vi "Vision_Processing_L_R9.vi"(0 "Current State":T2(ring), 1 "Image Dst":T6=refnum, 2 "Inpute Image":T6=refnum, 3 "Startup Flag":bool, 5 "Current ROI Descriptor":T11={"Global Rectangle"=[0, 0, 320, 220], "Contours"=[{"ID"=enum."External", "Type"=12, "Coordinates"=[0, 0, 320, 220, 0]}]} {"Contours"."Type" items=["No Selection", "Point", "Line", "Rectangle", "Oval", "Polygon", "Freehand Region", "Annulus", "Unused2", "Unused3", "Broken Line", "Freehand Line", "Rotated Rectangle"]}, 6 "Avg Score - Last":dbl=997.186962890625, 7 "error in (no error)":errorcluster, 8 "Current Settings":T9={"Curve Parameters"={"Extraction Mode"=1, "Edge Threshold"=150, "Edge Filter Size"=0, "Min Length"=15, "Row Search Step Size"=10, "Col Search Step Size"=10, "Max Endpoint Gap"=2, "Closed"=TRUE, "Subpixel"=TRUE}, "Match Mode"={"Rotation"=TRUE, "Scale"=TRUE, "Occlusion"=TRUE, "Reserved"=FALSE, "Reserved"=FALSE, "Reserved"=FALSE}, "Range Settings"=[{"Match Constraints"=0, "Min"=-5.0, "Max"=5.0}, {"Match Constraints"=1, "Min"=149.98635845184327, "Max"=172.71047382354737}, {"Match Constraints"=2, "Min"=0.0, "Max"=20.0}], "Number of Matches"=1, "Minimum Match Score"=900.0, "SubPixel Accuracy"=TRUE, "Adv. Geometric Match Options 2"=[{"Setup Data Item"=20, "Item Value"=0.0}, {"Setup Data Item"=22, "Item Value"=1.0}]} {"Curve Parameters"."Extraction Mode" items=["Normal", "Uniform Regions"]; "Curve Parameters"."Edge Filter Size" items=["Fine", "Normal", "Contour Tracing"]; "Curve Parameters"."Max Endpoint Gap" min=0; "Curve Parameters"."Col Search Step Size" min=1 max=255 step=1; "Curve Parameters"."Row Search Step Size" min=1 max=255 step=1; "Curve Parameters"."Min Length" min=0; "Curve Parameters"."Edge Threshold" min=1 max=350 step=1; "Range Settings"."Max" format="%.2f"; "Range Settings"."Min" format="%.2f"; "Range Settings"."Match Constraints" items=["Rotation Angle (degrees)", "Scale Factor (%)", "Occlusion (%)"]; "Adv. Geometric Match Options 2"."Setup Data Item" items=["Curve Extraction Mode", "Curve Edge Threshold", "Curve Edge Filter Size", "Min Curve Length", "Curve Row Search Step Size", "Curve Col Search Step Size", "Curve Max Endpoint Gap", "Extract Closed Curves", "Enable Subpixel Curve Extraction", "Enable Correlation Score", "Enable Subpixel Accuracy", "Subpixel Iterations", "Subpixel Tolerance", "Initial Match List Length", "Enable Target Template Curve Score", "Min Match Separation Distance", "Min Match Separation Angle", "Min Match Separation Scale", "Max Match Overlap", "Enable Coarse Result", "Enable Calibration Support", "Enable Contrast Reversal", "Search Strategy", "Refinement Match Factor", "Subpixel Match Factor"]}, 9 "Sub Beacon Search Enable":bool[](array[boolean])=[FALSE, FALSE, FALSE, FALSE, FALSE], 10 "History Data - IN":T5={"Valid Beacon History - in"=[TRUE, TRUE, TRUE, TRUE, TRUE, TRUE, TRUE, TRUE, TRUE, TRUE, TRUE, TRUE, TRUE, TRUE, TRUE, TRUE, TRUE, TRUE, TRUE, TRUE], "Valid Score History"=[996.9906616210938, 997.97216796875, 996.9906616210938, 996.9906616210938, 996.9906616210938, 996.9906616210938, 996.9906616210938, 996.9906616210938, 997.97216796875, 996.9906616210938, 996.9906616210938, 999.7824096679688, 999.7824096679688, 997.97216796875, 999.7824096679688, 999.7824096679688, 999.7824096679688, 999.7824096679688, 999.7824096679688, 999.7824096679688], "Valid Scale History"=[161.25363159179688, 161.6636962890625, 161.2349395751953, 161.27423095703125, 161.31558227539062, 160.97698974609375, 161.38648986816406, 161.37643432617188, 161.23867797851562, 161.21334838867188, 161.1531524658203, 161.44549560546875, 161.62496948242188, 161.1356201171875, 161.96054077148438, 161.54180908203125, 161.68902587890625, 161.53578186035156, 161.7397918701172, 161.8538360595703]} {"Valid Scale History" format="%#_13g"; "Valid Score History" format="%#_13g"}, 13 "Avg Scale - Last":dbl=161.34841613769532, 16 "History Size":i32=20) -> (11 "Avg Scale":dbl=161.34841613769532, 12 "Avg Score":dbl=997.186962890625, 14 "Tracking Info 1":T1={"Tracking Coordinates"={"X"=158.71055603027344, "Y"=95.56468963623047}, "Current Valid"=TRUE, "Current State - Out"=enum."Sub - 2", "Setting Values"={"Min Scale"=149.93676738739015, "Max Scale"=172.64940814971925, "Min Score"=900.0}}, 15 "Next Main ROI Descriptor":T3={"Global Rectangle"=[0, 0, 320, 220], "Contours"=[{"ID"=enum."External", "Type"=12, "Coordinates"=[0, 0, 320, 220, 0]}]} {"Contours"."Type" items=["No Selection", "Point", "Line", "Rectangle", "Oval", "Polygon", "Freehand Region", "Annulus", "Unused2", "Unused3", "Broken Line", "Freehand Line", "Rotated Rectangle"]}, 17 "Beacon - Scales":sgl[](array[numeric])=[163.2041, 163.79373, 0.0, 0.0, 0.0], 18 "History Data - Out":T4={"Valid Beacon History\nOut"=[TRUE, TRUE, TRUE, TRUE, TRUE, TRUE, TRUE, TRUE, TRUE, TRUE, TRUE, TRUE, TRUE, TRUE, TRUE, TRUE, TRUE, TRUE, TRUE, TRUE], "Valid Score History\nOut"=[996.9906616210938, 997.97216796875, 996.9906616210938, 996.9906616210938, 996.9906616210938, 996.9906616210938, 996.9906616210938, 996.9906616210938, 997.97216796875, 996.9906616210938, 996.9906616210938, 999.7824096679688, 999.7824096679688, 997.97216796875, 999.7824096679688, 999.7824096679688, 999.7824096679688, 999.7824096679688, 999.7824096679688, 999.7824096679688], "Valid Scale History\nOut"=[161.25363159179688, 161.6636962890625, 161.2349395751953, 161.27423095703125, 161.31558227539062, 160.97698974609375, 161.38648986816406, 161.37643432617188, 161.23867797851562, 161.21334838867188, 161.1531524658203, 161.44549560546875, 161.62496948242188, 161.1356201171875, 161.96054077148438, 161.54180908203125, 161.68902587890625, 161.53578186035156, 161.7397918701172, 161.8538360595703]} {"Valid Scale History\nOut" format="%#_13g"; "Valid Score History\nOut" format="%#_13g"}, 19 "Y Coordinates":sgl[](array[numeric])=[108.99595, 93.22681, 0.0, 0.0, 0.0], 20 "Beacons Found":bool[](array[boolean])=[TRUE, TRUE, FALSE, FALSE, FALSE], 21 "X Coordinates":sgl[](array[numeric])=[109.63992, 213.33662, 0.0, 0.0, 0.0], 22 "Next State":T2(ring), 23 "Lock Status":bool=TRUE, 24 "Startup Flag - out":bool, 25 "New Settings":T9={"Curve Parameters"={"Extraction Mode"=1, "Edge Threshold"=150, "Edge Filter Size"=0, "Min Length"=15, "Row Search Step Size"=10, "Col Search Step Size"=10, "Max Endpoint Gap"=2, "Closed"=TRUE, "Subpixel"=TRUE}, "Match Mode"={"Rotation"=TRUE, "Scale"=TRUE, "Occlusion"=TRUE, "Reserved"=FALSE, "Reserved"=FALSE, "Reserved"=FALSE}, "Range Settings"=[{"Match Constraints"=0, "Min"=-5.0, "Max"=5.0}, {"Match Constraints"=1, "Min"=149.98635845184327, "Max"=172.71047382354737}, {"Match Constraints"=2, "Min"=0.0, "Max"=20.0}], "Number of Matches"=1, "Minimum Match Score"=900.0, "SubPixel Accuracy"=TRUE, "Adv. Geometric Match Options 2"=[{"Setup Data Item"=20, "Item Value"=0.0}, {"Setup Data Item"=22, "Item Value"=1.0}]} {"Curve Parameters"."Extraction Mode" items=["Normal", "Uniform Regions"]; "Curve Parameters"."Edge Filter Size" items=["Fine", "Normal", "Contour Tracing"]; "Curve Parameters"."Max Endpoint Gap" min=0; "Curve Parameters"."Col Search Step Size" min=1 max=255 step=1; "Curve Parameters"."Row Search Step Size" min=1 max=255 step=1; "Curve Parameters"."Min Length" min=0; "Curve Parameters"."Edge Threshold" min=1 max=350 step=1; "Range Settings"."Max" format="%.2f"; "Range Settings"."Min" format="%.2f"; "Range Settings"."Match Constraints" items=["Rotation Angle (degrees)", "Scale Factor (%)", "Occlusion (%)"]}, 27 "Right Image 2":T6(plugin-control))   [LabVIEW 2015]
uses:
  <vilib>/vision/Image Controls.llb/IMAQ Image.ctl
  <vilib>/vision/Pattern Matching.llb/IMAQ Curve Parameters.ctl
  <vilib>/vision/Pattern Matching.llb/IMAQ Match Range Setting.ctl
panel:
  in  "ROBOT STATE(fwd, bwd, neither)":i32
  out "beacon - Scores":sgl[](array[numeric])=[998.9578, 999.6264, 0.0, 0.0, 0.0]
  in  "Minimum Score\nNormal 5":dbl=850.0
  in  "Minimum Score\nSub 4":dbl=850.0
  in  "Minimum Score\nSub 3":dbl=900.0
  in  "Minimum Score\nSub 2":dbl=900.0
  in  "Sub - 4 - FIle Path":path=path "/home/lvuser/natinst/bin/BeaconTemplates/4_beacons_left.png"
  in  "3 / 2\nTransition Scale":sgl=100.0
  in  "Score\nCushion- tight":dbl=75.0
  in  "Main ROI Decay\nper Fail (Vertical)":i32=5
  in  "ROI_factor(Horiztonal) (2 b)":sgl=2.0
  in  "ROI_factor(vertical) (2 b)":sgl=1.1
  in  "Sub - 2 File Path":path=path "/home/lvuser/natinst/bin/BeaconTemplates/2_beacons_left.png"
  out "Scale Decay \nFactor":dbl=11.36205768585205
  in  "Scale Decay \nFactor":dbl=5.0
  in  "Valid Treshold\nfor Lock":i16=3
  in  "Horiztonall Beacon \nCushion (pixels)":sgl=20.0
  out "New Min Score":dbl=900.0
  out "New Low Scale":dbl=149.98635845184327
  out "New high Scale":dbl=172.71047382354737
  in  "Absolute\nMinimum Score":dbl=800.0
  in  "Absolute\nMaximum Scale":dbl=300.0
  in  "Absolute\nMinimum Scale":dbl=10.0
  in  "Default No Lock\nSetting Values":T10={"Min Scale"=20.0, "Max Scale"=170.0, "Min Score"=800.0}
  in  "Score\nCushion":dbl=75.0
  out "Scale \nCushion":dbl=11.36205768585205
  in  "5 / 4\nTransition Scale":sgl=70.0
  in  "4 / 3\nTransition Scale":sgl=85.0
  in  "Timeout \nThrehsold":i32=1000
  in  "Main ROI Decay\nper Fail (Horiztonal)":i32=25
  in  "ROI_factor(Horiztonal) (4 & 5 b)":sgl=5.0
  in  "ROI_factor(vertical) (4 & 5 b)":sgl=1.5
  in  "ROI_factor(vertical) (3 b)":sgl=2.7
  in  "ROI_factor(Horiztonal) (3 b)":sgl=2.5
  out "Current  Score":sgl=996.99066
  out "Current  Scale":sgl=161.25363
  in  "Fail Count - In":i32
  in  "Sub Beacon Template File Path - ARRAY":path[](array[path])=[path "/home/lvuser/natinst/bin/BeaconTemplates/Sub1.png", path "/home/lvuser/natinst/bin/BeaconTemplates/Sub2.png", path "/home/lvuser/natinst/bin/BeaconTemplates/Sub3.png", path "/home/lvuser/natinst/bin/BeaconTemplates/Sub4.png", path "/home/lvuser/natinst/bin/BeaconTemplates/Sub5.png"]
  in  "Sub - 3 - FIle Path":path=path "/home/lvuser/natinst/bin/BeaconTemplates/3_beacons_left.png"
  in  "Normal - 5 - File Path":path=path "/home/lvuser/natinst/bin/BeaconTemplates/5_beacons.png"
  # "INPUTS"
  # "FILE PATHS"
  # "CONFIG"
  # "OUTPUTS"
  # "************"
  # "Range"
  # "Range"
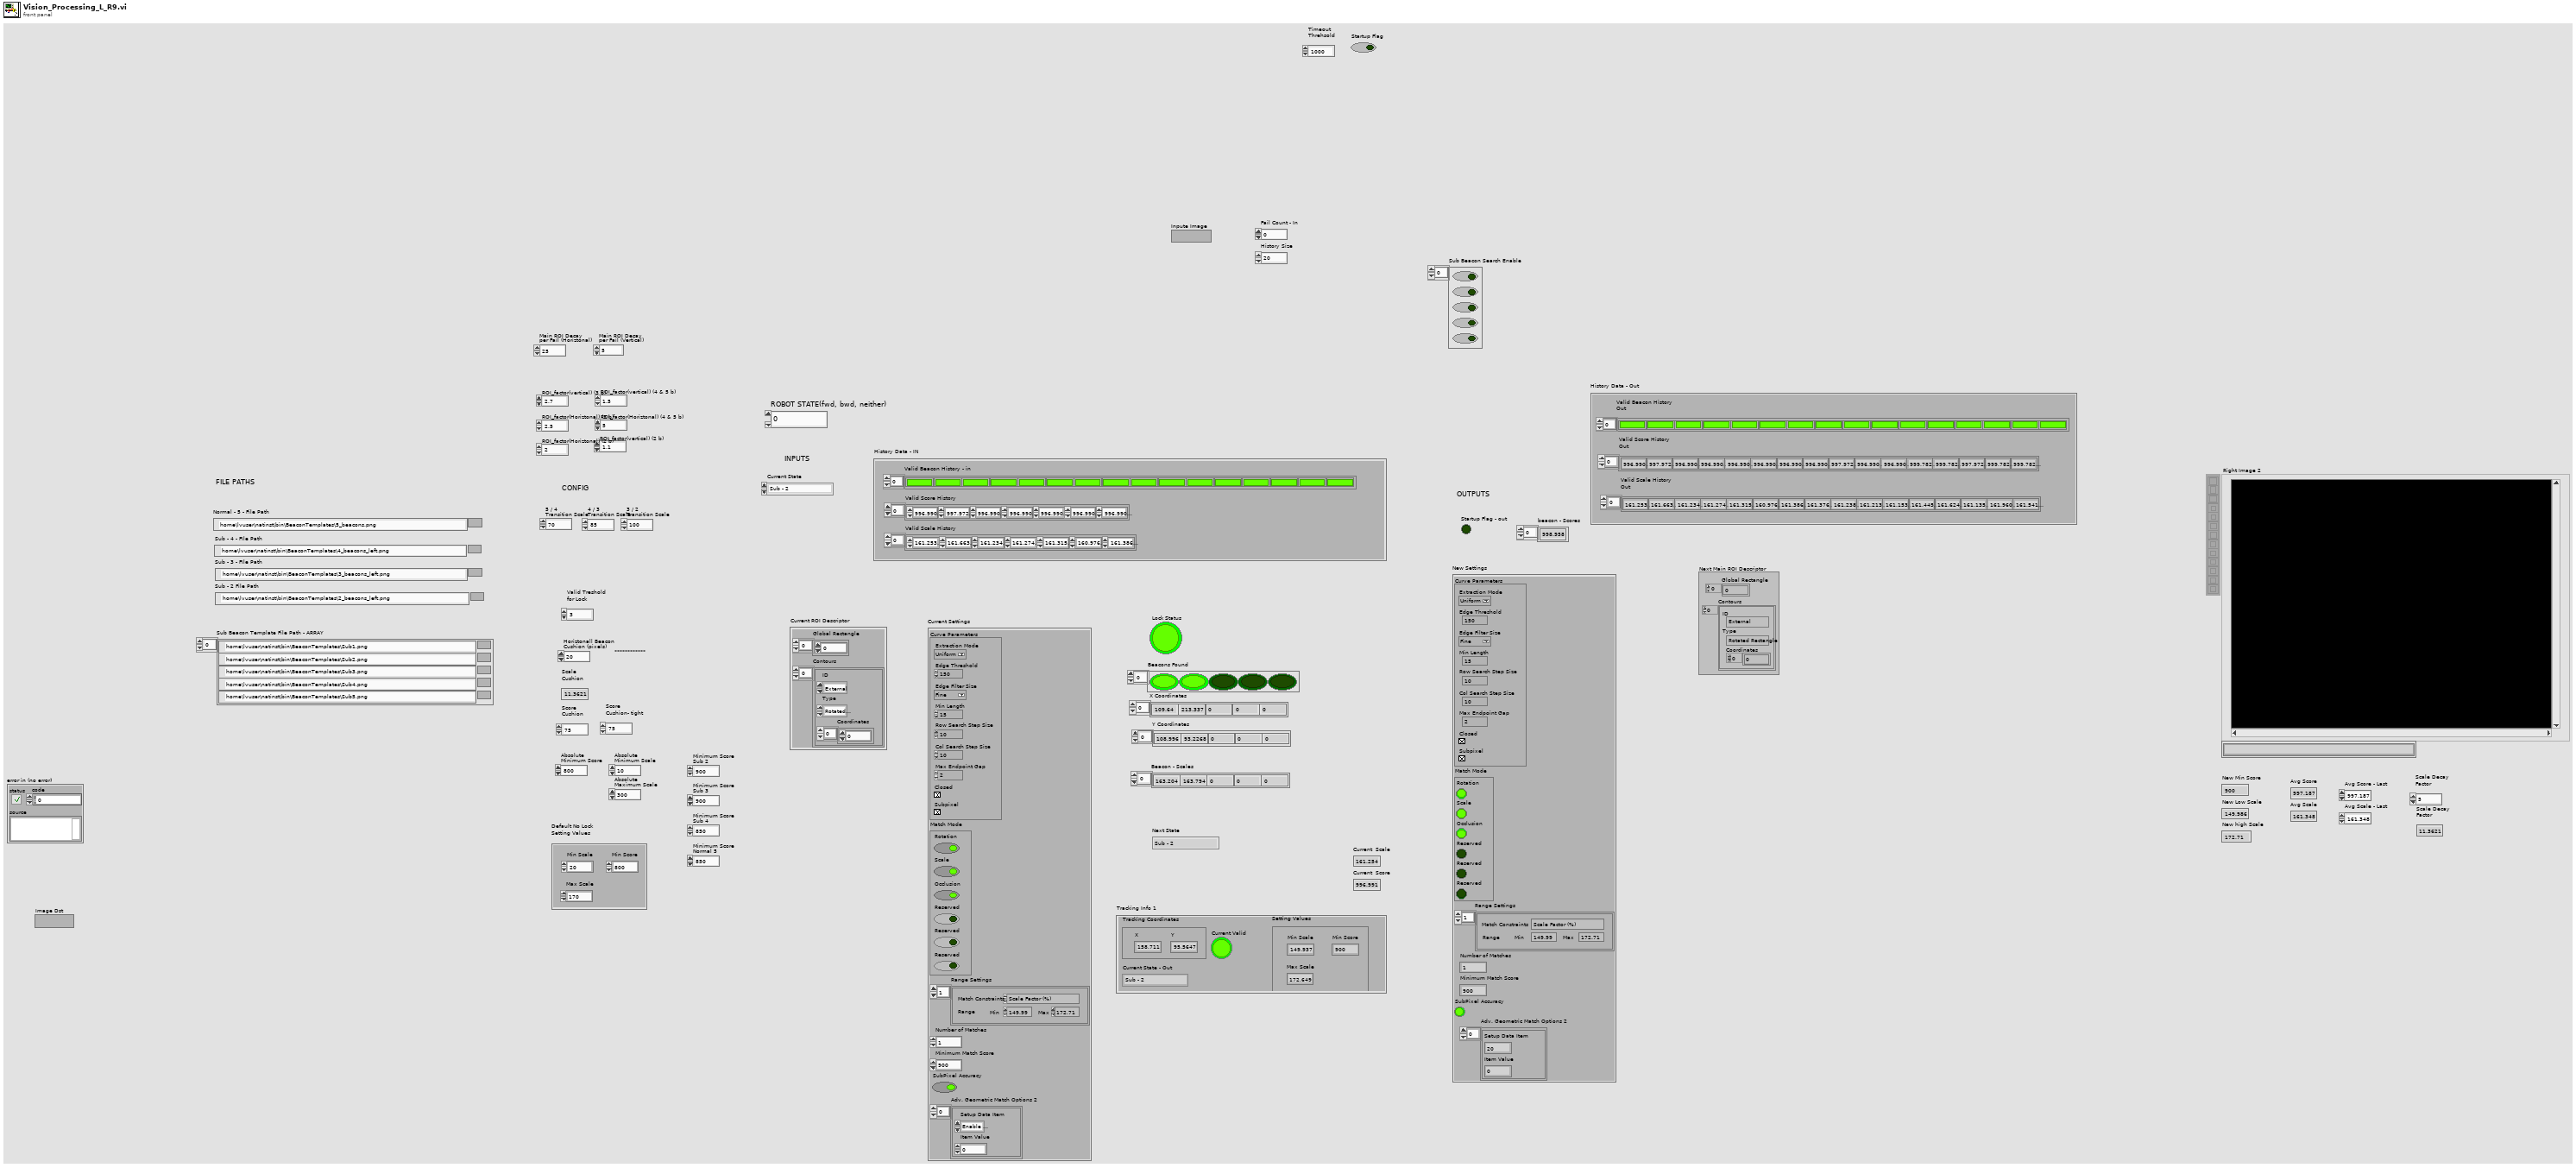
[diagram p1: front panel]
types:
  T1 = cluster{"Tracking Coordinates":cluster{"X":dbl, "Y":dbl}, "Current Valid":bool, "Current State - Out":enum16{"Sub - 2", "Sub - 3", "Sub - 4", "Normal - 5"}, "Setting Values":cluster{"Min Scale":dbl, "Max Scale":dbl, "Min Score":dbl}}
  T2 = enum16{"Sub - 2", "Sub - 3", "Sub - 4", "Normal - 5"}
  T3 = typedef "ROI Descriptor" = cluster{"Global Rectangle":i32[], "Contours":cluster{"ID":enum32{"External", "Internal"}, "Type":u32, "Coordinates":i32[]}[]}
  T4 = cluster{"Valid Beacon History\nOut":bool[], "Valid Score History\nOut":dbl[], "Valid Scale History\nOut":dbl[]}
  T5 = cluster{"Valid Beacon History - in":bool[], "Valid Score History":dbl[], "Valid Scale History":dbl[]}
  T6 = typedef "IMAQ Image.ctl" = refnum<image>
  T7 = typedef "IMAQ Curve Parameters.ctl" = cluster{"Extraction Mode":u32, "Edge Threshold":i32, "Edge Filter Size":u32, "Min Length":i32, "Row Search Step Size":i32, "Col Search Step Size":i32, "Max Endpoint Gap":i32, "Closed":bool, "Subpixel":bool}
  T8 = typedef "IMAQ Match Range Setting.ctl" = cluster{"Match Constraints":u32, "Min":dbl, "Max":dbl}
  T9 = cluster{"Curve Parameters":T7, "Match Mode":cluster{"Rotation":bool, "Scale":bool, "Occlusion":bool, "Reserved":bool, "Reserved":bool, "Reserved":bool}, "Range Settings":T8[], "Number of Matches":i32, "Minimum Match Score":sgl, "SubPixel Accuracy":bool, "Adv. Geometric Match Options 2":cluster{"Setup Data Item":u16, "Item Value":dbl}[]}
  T10 = cluster{"Min Scale":dbl, "Max Scale":dbl, "Min Score":dbl}
  T11 = cluster{"Global Rectangle":i32[], "Contours":cluster{"ID":enum32{"External", "Internal"}, "Type":u32, "Coordinates":i32[]}[]}
  T12 = typedef "IMAQ GM Match Report.ctl" = cluster{"Position":cluster{"x":sgl, "y":sgl}, "Angle":sgl, "Scale":sgl, "Score":sgl, "Bounding Box":cluster{"x":sgl, "y":sgl}[], "Contrast Reversed":bool, "Occlusion %":sgl, "Template Target Curve Score":sgl, "Target Template Curve Score":sgl, "Correlation Score":sgl}
  T13 = cluster{"Matches (Geometric Matching 1)[0]":T12, "Matches (Geometric Matching 1)[1]":T12, "Matches (Geometric Matching 1)[2]":T12, "Matches (Geometric Matching 1)[3]":T12, "Matches (Geometric Matching 1)[4]":T12, "Matches (Geometric Matching 1)[5]":T12, "Matches (Geometric Matching 1)[6]":T12, "Matches (Geometric Matching 1)[7]":T12, "Matches (Geometric Matching 1)[8]":T12}
  T14 = cluster{"Bounding Box[0]":cluster{"x":sgl, "y":sgl}, "Bounding Box[1]":cluster{"x":sgl, "y":sgl}, "Bounding Box[2]":cluster{"x":sgl, "y":sgl}, "Bounding Box[3]":cluster{"x":sgl, "y":sgl}, "Bounding Box[4]":cluster{"x":sgl, "y":sgl}, "Bounding Box[5]":cluster{"x":sgl, "y":sgl}, "Bounding Box[6]":cluster{"x":sgl, "y":sgl}, "Bounding Box[7]":cluster{"x":sgl, "y":sgl}, "Bounding Box[8]":cluster{"x":sgl, "y":sgl}}
  T15 = cluster{"index":u32, "Absolute\nMinimum Scale":dbl, "Absolute\nMaximum Scale":dbl}
  T16 = cluster{"New Low Scale":dbl, "New high Scale":dbl, "New Min Score":dbl}
  T17 = cluster{"Position":cluster{"x":sgl, "y":sgl}, bool, "Current State - Out":enum16{"Sub - 2", "Sub - 3", "Sub - 4", "Normal - 5"}, cluster{"New Low Scale":dbl, "New high Scale":dbl, "New Min Score":dbl}}
  T18 = cluster{"Position":cluster{"x":sgl, "y":sgl}, bool, "Current State":enum16{"Sub - 2", "Sub - 3", "Sub - 4", "Normal - 5"}, cluster{"New Low Scale":dbl, "New high Scale":dbl, "New Min Score":dbl}}
  T19 = typedef "IMAQ Rectangle" = cluster{"Left":i32, "Top":i32, "Right":i32, "Bottom":i32, "Rotation":dbl}
  T20 = cluster{"index":u32, "Min Scale":dbl, "Max Scale":dbl}
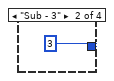
[diagram p3: hidden frame]
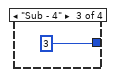
[diagram p4: hidden frame]
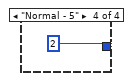
[diagram p5: hidden frame]
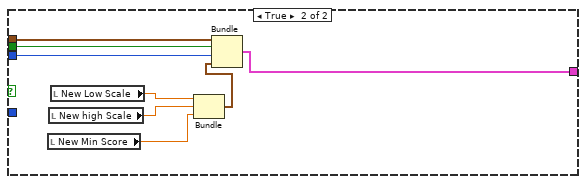
[diagram p6: hidden frame]
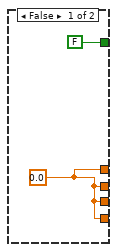
[diagram p7: hidden frame]
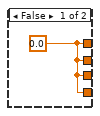
[diagram p8: hidden frame]
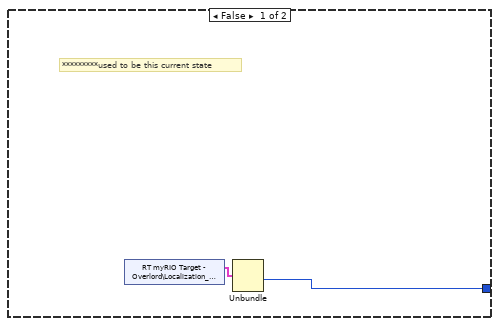
[diagram p12: hidden frame]
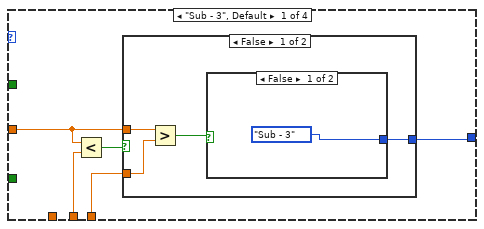
[diagram p13: hidden frame]
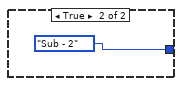
[diagram p14: hidden frame]
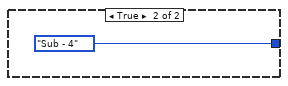
[diagram p15: hidden frame]
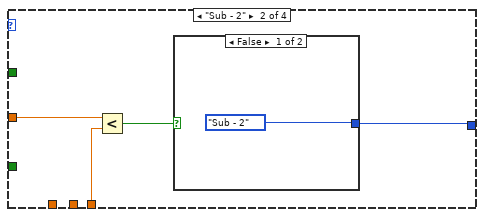
[diagram p16: hidden frame]
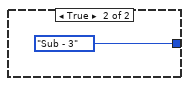
[diagram p17: hidden frame]
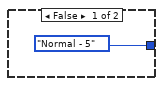
[diagram p18: hidden frame]
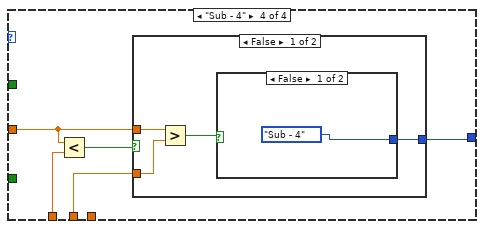
[diagram p19: hidden frame]
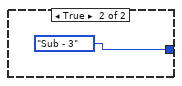
[diagram p20: hidden frame]
diagram:
  (unwired) enum16{"Short Range", "Long Range"}."Short Range"
  # "Next Settings"
  n1 = flat-sequence {
    tunnel: [w8] -> w3
    tunnel: [w7] -> w2
    tunnel: ["Image Dst"] -> w1
    tunnel: w3 -> [w157]
    tunnel: w2 -> [w155]
    tunnel: w1 -> [w156]
    frame #0 {
      # "APPLY FILTERING"
      n2 = call "Camera - Filtering"("Image In"="Inpute Image", "Image Dst"="Image Dst", "error in"="error in (no error)") -> ("Image Out"=w8:T6, "error out"=w7:errorcluster)  [unwired: 23 in]
    }
    frame #1 {
      w38 = u32 1 ("index")
      w119 = u32 1 ("index")
      w140 = u8 5
      # "*************************************************************************************************"
      # "Current Scale"
      # "Lower Scale"
      # "Upper Scale"
      # "Scale"
      # "Start up Template"
      # "Image Lock"
      # "Update Tracking Coordinates"
      # "CURRENT VALID"
      # "*************"
      # "Beacon - Y"
      # "Beacon - X"
      # "Beacons Found"
      # "Build ROI for Individual Beacons Based on Main Bounding Box"
      # "Starting X Lower Bound"
      # "Length of\nIndividual Beacon ROI"
      # "Length of Bounding Box"
      # "Choose ROI Factor based on Next State"
      # "Current Match"
      # "Current ROI"
      # "Image Lock"
      # "Force SR on Startup"
      # "Valid History"
      # "Draw ROI and stuff on outputi mage"
      # "Pull Down Startup IF Already True and Lock\nOtherwise don't update"
      # "Next Settings"
      # "Apply Limits to Settings"
      # "Scale"
      # "Min Score"
      # "Lower Scale"
      # "Upper Scale"
      # "Current Settings"
      # "Current Min\n& Max Scale"
      # "Current Valid"
      # "Update Search Settings"
      # "Update Template State"
      # "Calculate Average Scale/Score"
      # "max avg"
      # "Min Required to use avarage"
      # "Valid  Ccount\n(up to 3)"
      # "****# of previous in history that must be true\nin order for position to be considered \"locked\""
      # "Update Shift Arrays"
      # "# of Beacons Found to be valid"
      # "# of beacons"
      # "Matches"
      # "image out"
      n3 = Select(t=T2."Sub - 2", s="Startup Flag", f="Current State") -> (s? t:f=w47:T2)
      n4 = case shown="\"Sub - 4\"" w47 {
        tunnel: w157 -> [w537 w569 w600 w635]
        tunnel: w156 -> [w536 w568 w599 w634]
        tunnel: "Current ROI Descriptor" -> [w535 w567 w597 w633]
        tunnel: "Current Settings" -> [w534 w566 w596 w632]
        tunnel: [w530 w562 w593 w628] -> w83
        tunnel: [w529 w561 w594 w627] -> w103
        tunnel: [w527 w559 w595 w625] -> w148
        tunnel: w155 -> [_ _ w598 w624]
        tunnel: "Sub Beacon Search Enable" -> [w528 w560 w601 w623]
        tunnel: [sgl 3.0 ("y") sgl 2.0 ("y") 4.0 sgl 5.0 ("y")] -> w153
        tunnel: [w525 w557 w591 w621] -> w152
        tunnel: [2 2 3 4] -> w149
        frame "Sub - 3" {
          n5 = call "Short Range 2"("Image In"=w537, "Image Dst"=w536, "ROI Descriptor (Geometric Matching 1)"=w535, "Settings (Geometric Matching 1)"=w534, "Template File Path (Geometric Matching 1)"="Sub - 3 - FIle Path") -> ("Image Out"=w529:T6, "Matches (Geometric Matching 1)"=w530:T12[], "Number of Matches (Geometric Matching 1)"=w531:i32, "error out"=w525:errorcluster)  [unwired: 19 in]
          n6 = Equal?(x=w531, y=1) -> (x = y?=w532:bool)
          n7 = case shown="True" w532 {
            tunnel: w528 -> [w545 w548]
            tunnel: [w538 w549] -> w527
            frame False {
              w539 = FALSE
              # "F"
              # "No Main Found,\nDon't Search any Subs"
              n8 = Replace Array Subset(array=w545, new element #1=w539, index #1=0 ("y"), new element #2=w539, index #2=1 ("y"), new element #3=w539, index #3=2 ("y"), new element #4=w539, index #4=3 ("y"), new element #5=w539, index #5=4 ("y")) -> (w538:bool[])
            }
            frame True {
              w547 = TRUE
              w546 = FALSE
              n9 = Replace Array Subset(array=w548, new element #1=w547, index #1=0 ("y"), new element #2=w547, index #2=1 ("y"), new element #3=w547, index #3=2 ("y"), new element #4=w546, index #4=3 ("y"), new element #5=w546, index #5=4 ("y")) -> (w549:bool[])
            }
          }
        }
        frame "Sub - 2" {
          n10 = call "Short Range"("Image In"=w569, "Image Dst"=w568, "ROI Descriptor (Geometric Matching 1)"=w567, "Settings (Geometric Matching 1)"=w566, "Template File Path (Geometric Matching 1)"="Sub - 2 File Path") -> ("Image Out"=w561:T6, "Matches (Geometric Matching 1)"=w562:T12[], "Number of Matches (Geometric Matching 1)"=w563:i32, "error out"=w557:errorcluster)  [unwired: 19 in]
          n11 = Equal?(x=w563, y=1) -> (x = y?=w564:bool)
          n12 = case shown="True" w564 {
            tunnel: w560 -> [w577 w580]
            tunnel: [w570 w581] -> w559
            frame False {
              w571 = FALSE
              # "F"
              # "No Main Found,\nDon't Search any Subs"
              n13 = Replace Array Subset(array=w577, new element #1=w571, index #1=0 ("y"), new element #2=w571, index #2=1 ("y"), new element #3=w571, index #3=2 ("y"), new element #4=w571, index #4=3 ("y"), new element #5=w571, index #5=4 ("y")) -> (w570:bool[])
            }
            frame True {
              w579 = TRUE
              w578 = FALSE
              # "Search for specific Beacons"
              n14 = Replace Array Subset(array=w580, new element #1=w579, index #1=0 ("y"), new element #2=w579, index #2=1 ("y"), new element #3=w578, index #3=2 ("y"), new element #4=w578, index #4=3 ("y"), new element #5=w578, index #5=4 ("y")) -> (w581:bool[])
            }
          }
        }
        frame "Sub - 4" {
          # "**Make sure this selects the \nappropriate beacons to search for!!"
          n15 = call "Dumping Range"("Image In"=w600, "Image Dst"=w599, "ROI Descriptor (Geometric Matching 1)"=w597, "Settings (Geometric Matching 1)"=w596, "Template File Path (Geometric Matching 1)"="Sub - 4 - FIle Path", "error in"=w598) -> ("Image Out"=w594:T6, "Matches (Geometric Matching 1)"=w593:T12[], "Number of Matches (Geometric Matching 1)"=w590:i32, "error out"=w591:errorcluster)  [unwired: 18 in]
          n16 = Equal?(x=w590, y=1) -> (x = y?=w588:bool)
          n17 = case shown="True" w588 {
            tunnel: w601 -> [w610 w613]
            tunnel: [w603 w614] -> w595
            frame False {
              w604 = FALSE
              # "F"
              # "No Main Found,\nDon't Search any Subs"
              n18 = Replace Array Subset(array=w610, new element #1=w604, index #1=0 ("y"), new element #2=w604, index #2=1 ("y"), new element #3=w604, index #3=2 ("y"), new element #4=w604, index #4=3 ("y"), new element #5=w604, index #5=4 ("y")) -> (w603:bool[])
            }
            frame True {
              w612 = TRUE
              n19 = Replace Array Subset(array=w613, new element #1=w612, index #1=0 ("y"), new element #2=w612, index #2=1 ("y"), new element #3=w612, index #3=2 ("y"), new element #4=w612, index #4=3 ("y"), new element #5=FALSE, index #5=4 ("y")) -> (w614:bool[])
            }
          }
        }
        frame "Normal - 5" {
          n20 = call "Long Range"("Image In"=w635, "Image Dst"=w634, "ROI Descriptor (Geometric Matching 1)"=w633, "Settings (Geometric Matching 1)"=w632, "Template File Path (Geometric Matching 1)"="Normal - 5 - File Path", "error in"=w624) -> ("Image Out"=w627:T6, "Matches (Geometric Matching 1)"=w628:T12[], "Number of Matches (Geometric Matching 1)"=w630:i32, "error out"=w621:errorcluster)  [unwired: 18 in]
          n21 = Equal?(x=w630, y=1) -> (x = y?=w626:bool)
          n22 = case shown="True" w626 {
            tunnel: w623 -> [w643 w645]
            tunnel: [w636 w644] -> w625
            frame False {
              w637 = FALSE
              # "F"
              # "No Main Found,\nDon't Search any Subs"
              n23 = Replace Array Subset(array=w643, new element #1=w637, index #1=0 ("y"), new element #2=w637, index #2=1 ("y"), new element #3=w637, index #3=2 ("y"), new element #4=w637, index #4=3 ("y"), new element #5=w637, index #5=4 ("y")) -> (w636:bool[])
            }
            frame True {
              w646 = TRUE
              # "T"
              # "Search for ALL Beacons"
              n24 = Replace Array Subset(array=w645, new element #1=w646, index #1=0 ("y"), new element #2=w646, index #2=1 ("y"), new element #3=w646, index #3=2 ("y"), new element #4=w646, index #4=3 ("y"), new element #5=w646, index #5=4 ("y")) -> (w644:bool[])
            }
          }
        }
      }
      n25 = Array To Cluster(array=w83) -> (cluster=w73:T13)
      n26 = Unbundle By Name(w73) -> ("Matches (Geometric Matching 1)[0].Position"=w49:cluster{"x":sgl, "y":sgl}, "Matches (Geometric Matching 1)[0].Bounding Box"=w71:cluster{"x":sgl, "y":sgl}[], "Matches (Geometric Matching 1)[0].Scale"=w28:sgl, "Matches (Geometric Matching 1)[0].Score"=w110:sgl)
      "Current  Scale" <- w28
      "Current  Score" <- w110
      n27 = Array To Cluster(array=w71) -> (cluster=w72:T14)
      n28 = Unbundle By Name(w72) -> ("Bounding Box[0].x"=w62:sgl, "Bounding Box[0].y"=w61:sgl, "Bounding Box[2].x"=w60:sgl, "Bounding Box[2].y"=w59:sgl)
      n29 = Bundle("x"=w62, "y"=w61, "x"=w60, "y"=w59) -> (w57:cluster{"x":sgl, "y":sgl, "x":sgl, "y":sgl})  [unwired: 1 in]
      n30 = call "IMAQ Overlay Rectangle"("Rectangle"=w57, "Image"=w103) -> ("Image Out"=w58:T6)  [unwired: 8 in, 1 out]
      n31 = Subtract(x=w60, y=w62) -> (x-y=w66:sgl)
      n32 = Divide(x=w66, y=w153) -> (x/y=w68:dbl)
      n33 = Multiply(x="Horiztonall Beacon \nCushion (pixels)", y=w28) -> (x*y=w56:sgl)
      n34 = Divide(x=w56, y=sgl 100.0) -> (x/y=w53:sgl)
      n35 = Subtract(x=w61, y=w53) -> (x-y=w69:sgl)
      n36 = Add(x=w53, y=w59) -> (x+y=w70:sgl)
      n37 = for {
        N: 5 -> [_]
        tunnel: w148 -> [w248] mode=indexing
        shift-right: [w242] -> _
        shift-left: w62 -> [w247]
        tunnel: w68 -> [w246]
        tunnel: w69 -> [w239]
        tunnel: w70 -> [w238]
        tunnel: [w245] -> w64 mode=indexing
        tunnel: w53 -> [w240]
        # "Divide Bounding Box"
        # "Upper Bound of Current is\nLower Bound for Next"
        n38 = case shown="True" w248 {
          tunnel: w247 -> [w249 w250]
          tunnel: w246 -> [_ w252]
          tunnel: [w249 w251] -> w242
          tunnel: [w249 w250] -> w244
          frame False {
            # "Don't Care"
          }
          frame True {
            # "X Lower Bound"
            n39 = Add(x=w250, y=w252) -> (x+y=w251:dbl)
          }
        }
        n40 = Subtract(x=w244, y=w240) -> (x-y=w243:dbl)
        n41 = Add(x=w242, y=w240) -> (x+y=w241:dbl)
        n42 = call "Bound_RO_L_R0.vi"("Bottom Right - Y"=w238, "Right - X"=w241, "Top Left - Y"=w239, "Top  Left - x"=w243) -> ("ROI Descriptor"=w245:T3)  [unwired: 7 in]
      }
      n43 = local read "Absolute\nMaximum Scale"() -> (w29:dbl)
      n44 = local read "Absolute\nMinimum Scale"() -> (w30:dbl)
      n45 = local read "Scale \nCushion"() -> (w27:dbl)
      n46 = Add(x=w28, y=w27) -> (x+y=w25:dbl)
      n47 = Subtract(x=w28, y=w27) -> (x-y=w26:dbl)
      n48 = Less?(x=w26, y=w30) -> (x < y?=w34:bool)
      n49 = Greater?(x=w25, y=w29) -> (0:w31:bool)
      n50 = Greater?(x=w26, y=w25) -> (0:w35:bool)
      n51 = Less?(x=w25, y=w26) -> (x < y?=w32:bool)
      n52 = Or(x=w34, y=w35) -> (x .or. y?=w36:bool)
      n53 = Or(x=w31, y=w32) -> (x .or. y?=w33:bool)
      n54 = Select(t=w30, s=w36, f=w26) -> (s? t:f=w24:dbl)
      n55 = Select(t=w29, s=w33, f=w25) -> (s? t:f=w23:dbl)
      n56 = Unbundle By Name("Current Settings") -> ("Range Settings"=w19:T8[])
      n57 = Bundle("index"=w38, "Absolute\nMinimum Scale"=w24, "Absolute\nMaximum Scale"=w23) -> (w37:T15)  [unwired: 1 in]
      n58 = Replace Array Subset(array=w19, new element=w37, index=w38) -> (w22:T8[])
      n59 = Bundle By Name(cluster="Current Settings", "Range Settings"=w22) -> (w21:T9)
      n60 = for {
        N: 5 -> [_]
        tunnel: w103 -> [w215]
        tunnel: w152 -> [w214]
        tunnel: w64 -> [w207] mode=indexing
        tunnel: "Sub Beacon Template File Path - ARRAY" -> [w213] mode=indexing
        tunnel: [w212] -> w42 mode=indexing
        tunnel: [w211] -> w41 mode=indexing
        tunnel: [w210] -> w43 mode=indexing
        tunnel: w148 -> [w209] mode=indexing
        tunnel: w21 -> [w208]
        shift-right: [w205] -> w104
        shift-left: w58 -> [w206]
        tunnel: [w204] -> w94 mode=indexing
        tunnel: [w203] -> w12 mode=indexing
        n61 = case shown="True" w209 {
          tunnel: w215 -> [_ w230]
          tunnel: w214 -> [_ w229]
          tunnel: w207 -> [_ w228]
          tunnel: w213 -> [_ w227]
          tunnel: [w216 w223] -> w212
          tunnel: [w216 w222] -> w211
          tunnel: [FALSE w221] -> w210
          tunnel: w208 -> [_ w220]
          tunnel: [w216 w219] -> w204
          tunnel: [w216 w218] -> w203
          frame False {
            w216 = sgl 0.0 ("x")
          }
          frame True {
            n62 = call "Sub Beacon Pattern Match"("Image In"=w230, "ROI Descriptor (Geometric Matching 1)"=w228, "Settings (Geometric Matching 1)"=w220, "Template File Path (Geometric Matching 1)"=w227, "error in"=w229) -> ("Matches (Geometric Matching 1)"=w224:T12[], "Number of Matches (Geometric Matching 1)"=w225:i32)  [unwired: 19 in, 2 out]
            n63 = Equal?(x=w225, y=1) -> (x = y?=w221:bool)
            n64 = case shown="True" w221 {
              tunnel: w224 -> [_ w236]
              tunnel: [w231 w235] -> w223
              tunnel: [w231 w234] -> w222
              tunnel: [w231 w233] -> w219
              tunnel: [w231 w232] -> w218
              frame False {
                w231 = sgl 0.0 ("x")
              }
              frame True {
                n65 = Array To Cluster(array=w236) -> (cluster=w237:T13)
                n66 = Unbundle By Name(w237) -> ("Matches (Geometric Matching 1)[0].Position.x"=w235:sgl, "Matches (Geometric Matching 1)[0].Position.y"=w234:sgl, "Matches (Geometric Matching 1)[0].Scale"=w233:sgl, "Matches (Geometric Matching 1)[0].Score"=w232:sgl)
              }
            }
          }
        }
        n67 = call "IMAQ Overlay ROI"("ROI Descriptor"=w207, "Image"=w206) -> ("Image Out"=w205:T6)  [unwired: 8 in, 1 out]
      }
      "Beacons Found" <- w43
      "X Coordinates" <- w42
      "Y Coordinates" <- w41
      "Beacon - Scales" <- w94
      "beacon - Scores" <- w12
      n68 = Boolean To (0,1)(Boolean=w43) -> (0, 1=w150:i16[])
      n69 = Add Array Elements(numeric array=w150) -> (sum=w151:i16)
      n70 = Greater Or Equal?(x=w151, y=w149) -> (x >= y?=w48:bool)
      n71 = case shown="False" w48 {
        tunnel: "Fail Count - In" -> [w521 _]
        tunnel: [w520 u16 0] -> w133
        frame False {
          n72 = Increment(x=w521) -> (x+1=w520:i32)
        }
        frame True {
          # "reset fail count"
        }
      }
      n73 = Unbundle By Name("History Data - IN") -> ("Valid Beacon History - in"=w101:bool[], "Valid Score History"=w100:dbl[], "Valid Scale History"=w99:dbl[])
      n74 = Greater?(x=w133, y="Timeout \nThrehsold") -> (0:w50:bool)
      n75 = Decrement(x="History Size") -> (x-1=w146:i32)
      n76 = for {
        N: "History Size" -> [_]
        shift-right: [w498] -> w98
        shift-left: w101 -> [w486]
        tunnel: w146 -> [w494]
        shift-right: [w491] -> w97
        shift-left: w100 -> [w493]
        shift-right: [w490] -> w96
        shift-left: w99 -> [w492]
        tunnel: w110 -> [w489]
        tunnel: w28 -> [w488]
        tunnel: w48 -> [w487]
        i -> [w497]
        # "Reverse Index"
        n77 = Subtract(x=w494, y=w497) -> (x-y=w495:i32)
        n78 = Equal To 0?(x=w495) -> (x = 0?=w496:bool)
        n79 = case shown="True" w496 {
          tunnel: w495 -> [w499 w518]
          tunnel: w486 -> [w509 w511]
          tunnel: [w507 w510] -> w498
          tunnel: w487 -> [_ w519]
          tunnel: w493 -> [w504 w517]
          tunnel: w492 -> [w503 w516]
          tunnel: [w502 w514] -> w491
          tunnel: [w501 w515] -> w490
          tunnel: w489 -> [_ w513]
          tunnel: w488 -> [_ w512]
          frame False {
            # "Shift Old"
            n80 = Decrement(x=w499) -> (x-1=w500:i32)
            n81 = Index Array(array=w509, index=w500) -> (element=w508:bool)
            n82 = Index Array(array=w504, index=w500) -> (element=w506:dbl)
            n83 = Index Array(array=w503, index=w500) -> (element=w505:dbl)
            n84 = Replace Array Subset(array=w509, new element=w508, index=w499) -> (w507:bool[])
            n85 = Replace Array Subset(array=w504, new element=w506, index=w499) -> (w502:dbl[])
            n86 = Replace Array Subset(array=w503, new element=w505, index=w499) -> (w501:dbl[])
          }
          frame True {
            # "Scale"
            # "Score"
            # "Valid"
            # "insert New"
            n87 = Replace Array Subset(array=w517, new element=w513, index=w518) -> (w514:dbl[])
            n88 = Replace Array Subset(array=w516, new element=w512, index=w518) -> (w515:dbl[])
            n89 = Replace Array Subset(array=w511, new element=w519, index=w518) -> (w510:bool[])
          }
        }
      }
      n90 = Boolean To (0,1)(Boolean=w98) -> (0, 1=w144:i16[])
      n91 = Bundle("Valid Beacon History - in"=w98, "Valid Score History"=w97, "Valid Scale History"=w96) -> (→"History Data - Out":T5)  [unwired: 1 in]
      n92 = Add Array Elements(numeric array=w144) -> (sum=w145:i16)
      n93 = Greater Or Equal?(x=w145, y="Valid Treshold\nfor Lock") -> (x >= y?=w111:bool)
      "Lock Status" <- w111
      n94 = Initialize Array(u8 0, w140) -> (w142:u8[])
      n95 = while {
        shift-right: [w469] -> w138
        shift-left: w142 -> [w471]
        tunnel: w98 -> [w477] mode=indexing
        shift-right: [w475] -> w136
        shift-left: u8 0 -> [w478]
        tunnel: "History Size" -> [w476]
        tunnel: w140 -> [w468]
        i -> [w470]
        stop <- w472 stop-if-true
        # "Grab Last 2 Valid Indexes"
        n96 = case shown="True" w477 {
          tunnel: w478 -> [w480 w482]
          tunnel: [w480 w485] -> w475
          tunnel: w471 -> [w479 w484]
          tunnel: w470 -> [_ w483]
          tunnel: [w479 w481] -> w469
          frame False {
          }
          frame True {
            # "Update Index\nto use"
            # "Increment\nValid Count"
            n97 = Replace Array Subset(array=w484, new element=w483, index=w482) -> (w481:u8[])
            n98 = Increment(x=w482) -> (x+1=w485:u8)
          }
        }
        n99 = Greater?(x=w470, y=w476) -> (0:w473:bool)
        n100 = Greater Or Equal?(x=w475, y=w468) -> (x >= y?=w474:bool)
        n101 = Or(x=w474, y=w473) -> (x .or. y?=w472:bool)
      }
      n102 = Greater?(x=w136, y=u8 2) -> (0:w137:bool)
      n103 = case shown="False" w137 {
        tunnel: w136 -> [_ w452]
        tunnel: w138 -> [_ w458]
        tunnel: w97 -> [_ w457]
        tunnel: w96 -> [_ w456]
        tunnel: ["Avg Score - Last" w450] -> w108
        tunnel: ["Avg Scale - Last" w449] -> w14
        frame False {
        }
        frame True {
          w455 = 0.0
          n104 = for {
            N: w452 -> [_]
            tunnel: w458 -> [w465] mode=indexing
            tunnel: w457 -> [w467]
            tunnel: w456 -> [w466]
            shift-right: [w463] -> w454
            shift-left: w455 -> [w461]
            shift-right: [w464] -> w453
            shift-left: w455 -> [w460]
            # "Fetch Last Valid Values"
            n105 = Index Array(array=w467, index=w465) -> (element=w462:dbl)
            n106 = Index Array(array=w466, index=w465) -> (element=w459:dbl)
            n107 = Add(x=w462, y=w461) -> (x+y=w463:dbl)
            n108 = Add(x=w459, y=w460) -> (x+y=w464:dbl)
          }
          n109 = To Double Precision Float(number=w452) -> (double precision float=w451:dbl)
          n110 = Divide(x=w454, y=w451) -> (x/y=w450:dbl)
          n111 = Divide(x=w453, y=w451) -> (x/y=w449:dbl)
        }
      }
      "Avg Score" <- w108
      "Avg Scale" <- w14
      n112 = case shown="True" w111 {
        tunnel: w50 -> [_ w270]
        tunnel: "4 / 3\nTransition Scale" -> [_ w269]
        tunnel: "5 / 4\nTransition Scale" -> [_ w268]
        tunnel: w14 -> [_ w267]
        tunnel: w111 -> [_ w266]
        tunnel: [w262 w265] -> w39
        tunnel: "3 / 2\nTransition Scale" -> [_ w264]
        frame False {
          # "*********used to be this current state"
          n113 = shared-variable "RT myRIO Target - Overlord\\Localization_Variables_r0.lvlib\\Info - Right"() -> (w263:T1)  [unwired: 1 in, 1 out]
          n114 = Unbundle(w263) -> ("Current State - Out"=w262:T2)  [unwired: 3 out]
        }
        frame True {
          # "Timeout"
          n115 = local read "Current State"() -> (w271:T2)
          n116 = case shown="\"Normal - 5\"" w271 {
            tunnel: w266 -> [_ _ _ _]
            tunnel: w267 -> [w275 w287 w292 w298]
            tunnel: w270 -> [_ _ _ _]
            tunnel: w269 -> [w276 _ _ w297]
            tunnel: w268 -> [_ _ w291 w300]
            tunnel: [w272 w284 w290 w296] -> w265
            tunnel: w264 -> [w273 w286 _ _]
            frame "Sub - 3", Default {
              n117 = Less?(x=w275, y=w276) -> (x < y?=w274:bool)
              n118 = case shown="False" w274 {
                tunnel: w275 -> [w280 _]
                tunnel: [w277 T2."Sub - 4"] -> w272
                tunnel: w273 -> [w279 _]
                frame False {
                  n119 = Greater?(x=w280, y=w279) -> (0:w278:bool)
                  n120 = case shown="False" w278 {
                    tunnel: [T2."Sub - 3" T2."Sub - 2"] -> w277
                    frame False {
                    }
                    frame True {
                    }
                  }
                }
                frame True {
                }
              }
            }
            frame "Sub - 2" {
              n121 = Less?(x=w287, y=w286) -> (x < y?=w285:bool)
              n122 = case shown="False" w285 {
                tunnel: [T2."Sub - 2" T2."Sub - 3"] -> w284
                frame False {
                }
                frame True {
                }
              }
            }
            frame "Normal - 5" {
              # "If Out of Scale Range\nor Timeout"
              n123 = Greater?(x=w292, y=w291) -> (0:w293:bool)
              n124 = case shown="True" w293 {
                tunnel: [T2."Normal - 5" T2."Sub - 4"] -> w290
                frame False {
                }
                frame True {
                }
              }
            }
            frame "Sub - 4" {
              n125 = Less?(x=w298, y=w300) -> (x < y?=w299:bool)
              n126 = case shown="False" w299 {
                tunnel: w298 -> [w304 _]
                tunnel: [w301 T2."Normal - 5"] -> w296
                tunnel: w297 -> [w303 _]
                frame False {
                  n127 = Greater?(x=w304, y=w303) -> (0:w302:bool)
                  n128 = case shown="False" w302 {
                    tunnel: [T2."Sub - 4" T2."Sub - 3"] -> w301
                    frame False {
                    }
                    frame True {
                    }
                  }
                }
                frame True {
                }
              }
            }
          }
        }
      }
      "Next State" <- w39
      n129 = local read "Current State"() -> (w44:T2)
      n130 = Equal?(x=w44, y=w39) -> (x = y?=w40:bool)
      n131 = case shown="False" w40 {
        tunnel: w49 -> [w167 w202]
        tunnel: w48 -> [w164 w201]
        tunnel: w47 -> [_ w200]
        tunnel: [w163 w199] -> w11
        tunnel: w39 -> [w161 _]
        tunnel: w43 -> [w171 _]
        tunnel: w42 -> [w169 _]
        tunnel: w41 -> [w168 _]
        frame False {
          # "Beacon Index"
          # "Check if Tracking is Available for the Next Template State"
          n132 = case shown="\"Sub - 2\", Default" w161 {
            tunnel: [4 3 3 2] -> w166
            frame "Sub - 2", Default {
            }
            frame "Sub - 3" {
            }
            frame "Sub - 4" {
            }
            frame "Normal - 5" {
            }
          }
          n133 = Index Array(array=w171, index=w166) -> (element=w170:bool)
          n134 = case shown="True" w170 {
            tunnel: w169 -> [_ w190]
            tunnel: w168 -> [_ w189]
            tunnel: [w172 w186] -> w165
            tunnel: w167 -> [w172 w187]
            tunnel: w166 -> [_ w188]
            frame False {
            }
            frame True {
              w183 = sgl 0.4 ("y")
              n135 = Unbundle(w187) -> ("x"=w184:sgl, "y"=w182:sgl)
              n136 = Index Array(array=w190, index=w188) -> (element=w179:sgl)
              n137 = Index Array(array=w189, index=w188) -> (element=w180:sgl)
              n138 = Subtract(x=sgl 1.0, y=w183) -> (x-y=w181:sgl)
              n139 = Multiply(x=w181, y=w179) -> (x*y=w177:sgl)
              n140 = Multiply(x=w181, y=w180) -> (x*y=w175:sgl)
              n141 = Multiply(x=w183, y=w184) -> (x*y=w178:sgl)
              n142 = Multiply(x=w183, y=w182) -> (x*y=w176:sgl)
              n143 = Add(x=w178, y=w177) -> (x+y=w174:sgl)
              n144 = Add(x=w176, y=w175) -> (x+y=w173:sgl)
              n145 = Bundle(w174, w173) -> (w186:cluster{sgl, sgl})  [unwired: 1 in]
            }
          }
          n146 = local read "New Min Score"() -> (w158:dbl)
          n147 = local read "New high Scale"() -> (w159:dbl)
          n148 = local read "New Low Scale"() -> (w160:dbl)
          n149 = Bundle("New Low Scale"=w160, "New high Scale"=w159, "New Min Score"=w158) -> (w162:T16)  [unwired: 1 in]
          n150 = Bundle("Position"=w165, w164, "Current State - Out"=w161, w162) -> (w163:T17)  [unwired: 1 in]
        }
        frame True {
          n151 = local read "New Min Score"() -> (w196:dbl)
          n152 = local read "New high Scale"() -> (w197:dbl)
          n153 = local read "New Low Scale"() -> (w198:dbl)
          n154 = Bundle("New Low Scale"=w198, "New high Scale"=w197, "New Min Score"=w196) -> (w195:T16)  [unwired: 1 in]
          n155 = Bundle("Position"=w202, w201, "Current State"=w200, w195) -> (w199:T18)  [unwired: 1 in]
        }
      }
      "Tracking Info 1" <- w11
      n156 = Unbundle By Name("Current Settings") -> ("Minimum Match Score"=w130:sgl, "Range Settings"=w116:T8[])
      n157 = case shown="\"Sub - 4\", Default" w39 {
        tunnel: "ROI_factor(vertical) (3 b)" -> [_ _ w261]
        tunnel: "ROI_factor(Horiztonal) (3 b)" -> [_ _ w260]
        tunnel: "ROI_factor(vertical) (4 & 5 b)" -> [_ w258 _]
        tunnel: "ROI_factor(Horiztonal) (4 & 5 b)" -> [_ w257 _]
        tunnel: "ROI_factor(vertical) (2 b)" -> [w255 _ _]
        tunnel: "ROI_factor(Horiztonal) (2 b)" -> [w254 _ _]
        tunnel: [w255 w258 w261] -> w76
        tunnel: [w254 w257 w260] -> w75
        tunnel: "Minimum Score\nSub 2" -> [w253 _ _]
        tunnel: [w253 w256 w259] -> w15
        tunnel: "Minimum Score\nSub 3" -> [_ _ w259]
        tunnel: "Minimum Score\nSub 4" -> [_ w256 _]
        frame "Sub - 2" {
        }
        frame "Sub - 4", Default {
        }
        frame "Sub - 3" {
        }
      }
      n158 = Index Array(array=w116, index=u32 1) -> (element=w129:T8)
      n159 = Unbundle(w129) -> ("Min"=w127:dbl, "Max"=w126:dbl)  [unwired: 1 out]
      n160 = And(x="Startup Flag", y=w111) -> (x .and. y?=w114:bool)
      n161 = case shown="True" w114 {
        tunnel: "Startup Flag" -> [w308 _]
        tunnel: [w308 FALSE] -> w113
        frame False {
        }
        frame True {
        }
      }
      "Startup Flag - out" <- w113
      n162 = call "Scaling and Mapping"("Signals"=w14) -> ("Scaled Signals"=w13:dynamicdata)  [unwired: 9 in, 1 out]
      n163 = To Single Precision Float(number=w13) -> (single precision float=w9:sgl)
      "Scale \nCushion" <- w9
      "Scale Decay \nFactor" <- w9
      n164 = case shown="True" w111 {
        tunnel: w48 -> [_ w368]
        tunnel: w108 -> [w322 w367]
        tunnel: w14 -> [w321 w366]
        tunnel: w130 -> [_ w365]
        tunnel: w127 -> [_ w364]
        tunnel: w126 -> [_ w363]
        tunnel: [w312 w342] -> w117
        tunnel: [w310 w354] -> w87
        tunnel: [w311 w353] -> w88
        tunnel: w9 -> [w324 w362]
        tunnel: "Score\nCushion" -> [w323 w361]
        tunnel: "Scale Decay \nFactor" -> [_ w360]
        tunnel: w9 -> [_ w359]
        tunnel: "Current ROI Descriptor" -> [_ w355]
        tunnel: w83 -> [_ w356]
        tunnel: w76 -> [_ w358]
        tunnel: w75 -> [_ w357]
        tunnel: [w314 w352] -> w74
        tunnel: w40 -> [_ w347]
        tunnel: w39 -> [_ w346]
        tunnel: w15 -> [_ w343]
        tunnel: "ROBOT STATE(fwd, bwd, neither)" -> [_ w341]
        tunnel: w9 -> [_ w340]
        frame False {
          # "Check Lock Status of OTHER Cam,\n\nif True,\n\nthen use it's settings,\n\notherwise use default no lock"
          # "Initial ROI Descriptor"
          # "Apply No Lock Default for each Template"
          n165 = disable-structure shown="Disabled" {
            disable-tunnel: [w339 _] -> _
            disable-tunnel: [w338 _] -> _
            disable-tunnel: w324 -> [w337 _]
            disable-tunnel: w323 -> [w336 _]
            disable-tunnel: w322 -> [w335 _]
            disable-tunnel: w321 -> [w334 _]
            frame Disabled {
              n166 = Subtract(x=w335, y=w336) -> ()  [unwired: 1 out]
              n167 = Subtract(x=w334, y=w337) -> (x-y=w339:dbl)
              n168 = Add(x=w337, y=w334) -> (x+y=w338:dbl)
            }
            frame Enabled {
            }
          }
          n169 = shared-variable "RT myRIO Target - Overlord\\Localization_Variables_r0.lvlib\\Image Lock - R"() -> (w313:bool)  [unwired: 1 in, 1 out]
          n170 = case shown="True" w313 {
            tunnel: [w327 w331] -> w312
            tunnel: [w325 w330] -> w311
            tunnel: [w326 w329] -> w310
            frame False {
              n171 = Unbundle By Name("Default No Lock\nSetting Values") -> ("Min Score"=w327:dbl, "Min Scale"=w326:dbl, "Max Scale"=w325:dbl)
            }
            frame True {
              n172 = shared-variable "RT myRIO Target - Overlord\\Localization_Variables_r0.lvlib\\Info - Right"() -> (w333:T1)  [unwired: 1 in, 1 out]
              n173 = Unbundle(w333) -> ("Setting Values"=w332:T10)  [unwired: 3 out]
              n174 = Unbundle(w332) -> ("Min Scale"=w329:dbl, "Max Scale"=w330:dbl, "Min Score"=w331:dbl)
            }
          }
          n175 = Bundle(0, 0, 640, 480, 0) -> (w320:cluster{i32, i32, i32, i32, i32})  [unwired: 1 in]
          n176 = call "IMAQ Convert Rectangle to ROI"("Rectangle"=w320) -> ("ROI Descriptor"=w314:T3)  [unwired: 8 in, 1 out]
        }
        frame True {
          # "Score out"
          # "Apply Limits to ROI"
          n177 = case shown="False" w368 {
            tunnel: w367 -> [_ w418]
            tunnel: [w386 w415] -> w344
            tunnel: w366 -> [_ w417]
            tunnel: [w385 w397] -> w354
            tunnel: [w384 w396] -> w353
            tunnel: w364 -> [w391 _]
            tunnel: w363 -> [w390 _]
            tunnel: w365 -> [w389 _]
            tunnel: w362 -> [_ w399]
            tunnel: w361 -> [_ w416]
            tunnel: w360 -> [w388 _]
            tunnel: w359 -> [w387 _]
            tunnel: w358 -> [_ w406]
            tunnel: w357 -> [_ w405]
            tunnel: w356 -> [_ w404]
            tunnel: [w377 w395] -> w351
            tunnel: [w376 w403] -> w350
            tunnel: [w375 w394] -> w349
            tunnel: [w374 w402] -> w348
            tunnel: w355 -> [w382 _]
            tunnel: w347 -> [_ _]
            tunnel: w346 -> [_ w401]
            tunnel: w341 -> [_ w392]
            tunnel: w340 -> [w370 _]
            frame False {
              # "Decrement Score by"
              n178 = Subtract(x=w391, y=w387) -> (x-y=w385:dbl)
              n179 = Add(x=w387, y=w390) -> (x+y=w384:dbl)
              n180 = Subtract(x=w389, y=w388) -> (x-y=w386:dbl)
              n181 = call "IMAQ Convert ROI to Rectangle"("ROI Descriptor"=w382) -> ("Rectangle"=w383:T19)  [unwired: 8 in, 1 out]
              n182 = Unbundle By Name(w383) -> ("Left"=w381:i32, "Top"=w380:i32, "Right"=w379:i32, "Bottom"=w378:i32)
              n183 = Divide(x=w370, y=sgl 3.0) -> (x/y=w369:sgl)
              n184 = To Long Integer(number=w370) -> (32bit integer=w372:i32)
              n185 = To Long Integer(number=w369) -> (32bit integer=w373:i32)
              n186 = Subtract(x=w381, y=w372) -> (x-y=w377:i32)
              n187 = Add(x=w379, y=w372) -> (x+y=w375:i32)
              n188 = Add(x=w378, y=w373) -> (x+y=w374:i32)
              n189 = Subtract(x=w380, y=w373) -> (x-y=w376:i32)
            }
            frame True {
              # "****"
              # "if switching states"
              # "Scale / Score"
              # "Main ROI"
              # "Horizontal Scale \n(smaller number = smaller ROI)"
              n190 = case shown="-1" w392 {
                tunnel: w417 -> [w422 w427 w432]
                tunnel: [w421 w423 w428] -> w400
                tunnel: w399 -> [w420 w426 w431]
                tunnel: [w419 w424 w429] -> w398
                frame 0, Default {
                  n191 = Subtract(x=w422, y=w420) -> (x-y=w419:dbl)
                  n192 = Add(x=w420, y=w422) -> (x+y=w421:dbl)
                }
                frame 1 {
                  n193 = Subtract(x=w427, y=5.0) -> (x-y=w424:dbl)
                  n194 = Add(x=w426, y=w427) -> (x+y=w423:dbl)
                }
                frame -1 {
                  n195 = Subtract(x=w432, y=w431) -> (x-y=w429:dbl)
                  n196 = Add(x=5.0 ("y"), y=w432) -> (x+y=w428:dbl)
                }
              }
              n197 = Subtract(x=w418, y=w416) -> (x-y=w415:dbl)
              n198 = Array To Cluster(array=w404) -> (cluster=w414:T13)
              n199 = Unbundle By Name(w414) -> ("Matches (Geometric Matching 1)[0].Position.x"=w408:sgl, "Matches (Geometric Matching 1)[0].Position.y"=w410:sgl, "Matches (Geometric Matching 1)[0].Scale"=w409:sgl)
              n200 = Divide(x=w409, y=w406) -> (x/y=w411:sgl)
              n201 = Multiply(x=w409, y=w405) -> (x*y=w413:sgl)
              n202 = Divide(x=w413, y=sgl 2.0) -> (x/y=w407:sgl)
              n203 = Add(x=w410, y=w411) -> (x+y=w402:sgl)
              n204 = Subtract(x=w410, y=w411) -> (x-y=w403:sgl)
              n205 = Subtract(x=w408, y=w407) -> (x-y=w395:sgl)
              n206 = Add(x=w407, y=w408) -> (x+y=w394:sgl)
              n207 = case shown="False" FALSE {
                tunnel: w401 -> [_ _]
                tunnel: [w435 w444] -> w396
                tunnel: w400 -> [w435 w446]
                tunnel: [w436 w443] -> w397
                tunnel: w398 -> [w436 w445]
                tunnel: w399 -> [_ w442]
                tunnel: [w434 w439] -> _
                tunnel: w395 -> [w434 w440]
                tunnel: [w433 w438] -> _
                tunnel: w394 -> [w433 w441]
                frame False {
                }
                frame True {
                  w437 = sgl 50.0 ("y")
                  # "Double scale cushion\nif changing states"
                  n208 = Add(x=w446, y=w442) -> (x+y=w444:dbl)
                  n209 = Subtract(x=w445, y=w442) -> (x-y=w443:dbl)
                  n210 = Subtract(x=w440, y=w437) -> (x-y=w439:sgl)
                  n211 = Add(x=w437, y=w441) -> (x+y=w438:sgl)
                }
              }
            }
          }
          n212 = Less?(x=w344, y=w343) -> (x < y?=w345:bool)
          n213 = call "Bound_RO_L_R0.vi"("Bottom Right - Y"=w348, "Right - X"=w349, "Top Left - Y"=w350, "Top  Left - x"=w351) -> ("ROI Descriptor"=w352:T3)  [unwired: 7 in]
          n214 = Select(t=w344, s=w345, f=w343) -> (s? t:f=w342:dbl)
        }
      }
      "Next Main ROI Descriptor" <- w74
      n215 = Less?(x=w117, y="Absolute\nMinimum Score") -> (x < y?=w121:bool)
      n216 = Less?(x=w87, y="Absolute\nMinimum Scale") -> (x < y?=w90:bool)
      n217 = Greater?(x=w88, y="Absolute\nMaximum Scale") -> (0:w85:bool)
      n218 = Greater?(x=w87, y=w88) -> (0:w91:bool)
      n219 = Less?(x=w88, y=w87) -> (x < y?=w86:bool)
      n220 = Select(t="Absolute\nMinimum Score", s=w121, f=w117) -> (s? t:f=w123:dbl)
      "New Min Score" <- w123
      n221 = Or(x=w90, y=w91) -> (x .or. y?=w92:bool)
      n222 = Or(x=w85, y=w86) -> (x .or. y?=w89:bool)
      n223 = Select(t="Absolute\nMinimum Scale", s=w92, f=w87) -> (s? t:f=w105:dbl)
      "New Low Scale" <- w105
      n224 = Select(t="Absolute\nMaximum Scale", s=w89, f=w88) -> (s? t:f=w106:dbl)
      "New high Scale" <- w106
      n225 = Bundle("index"=w119, "Min Scale"=w105, "Max Scale"=w106) -> (w118:T20)  [unwired: 1 in]
      n226 = Replace Array Subset(array=w116, new element=w118, index=w119) -> (w120:T8[])
      n227 = call "IMAQ Overlay ROI"("ROI Descriptor"=w74, "Image"=w104) -> ("Image Out"=→"Right Image 2":T6)  [unwired: 8 in, 1 out]
      n228 = Bundle By Name(cluster="Current Settings", "Range Settings"=w120, "Minimum Match Score"=w123) -> (→"New Settings":T9)
    }
  }
